vi "Dispose.vi"(8 "error in (no error)":errorcluster, 11 "ConcreteProductB":refnum<class "ConcreteProductB.lvclass">) -> (0 "error out":errorcluster)   [LabVIEW 2020, in "FactoryMethod.lvlib" / "ConcreteProductB.lvclass"]
uses:
  ConcreteProductB.lvclass
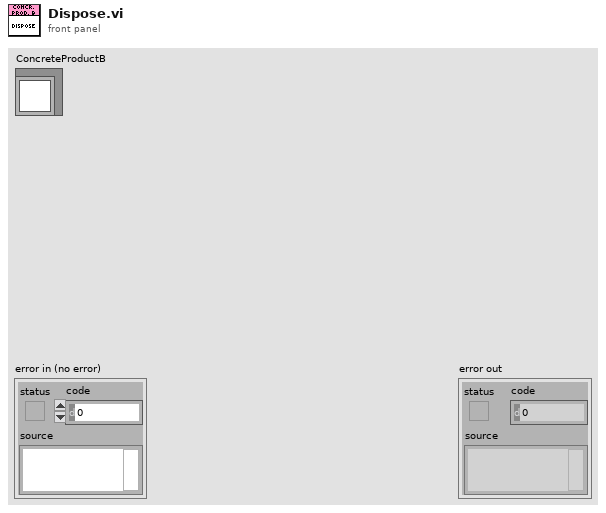
[diagram p1: front panel]
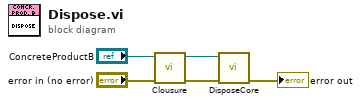
[diagram p0: block diagram]
diagram:
  n1 = call-dynamic "Clousure.vi"("error in (no error)"="error in (no error)", "ConcreteProductB in"="ConcreteProductB") -> ("error out"=w3:errorcluster, "ConcreteProductB out"=w2:refnum<class "ConcreteProductB.lvclass">)  [unwired: 8 in]
  n2 = call-dynamic "DisposeCore.vi"("error in (no error)"=w3, "ConcreteProductA in"=w2) -> ("error out"=→"error out":errorcluster)  [unwired: 8 in, 1 out]
